vi "Default Settings.vi"(8 "error in (no error)":errorcluster, 11 "CAD Dispense in":refnum<class "CAD Dispense.lvclass">) -> (0 "error out":errorcluster, 3 "CAD Dispense out":refnum<class "CAD Dispense.lvclass">)   [LabVIEW 2020, in "CAD Dispense.lvclass"]
uses:
  CAD Dispense.lvclass
panel:
  # "This Routine does not Accept Settings"
  # "This Routine Does not Accept Settings"
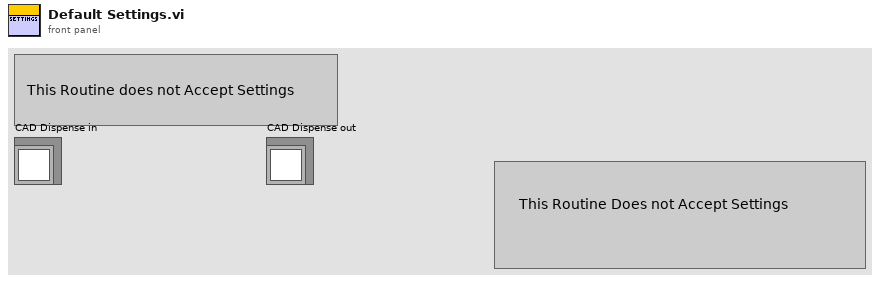
[diagram p1: front panel]
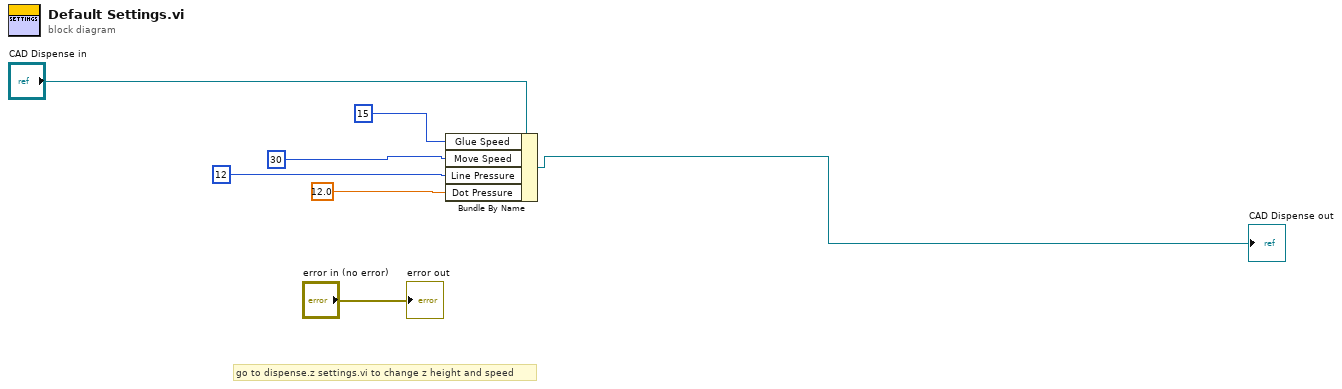
[diagram p0: block diagram]
diagram:
  # "go to dispense.z settings.vi to change z height and speed"
  n1 = Bundle By Name(cluster="CAD Dispense in", "Glue Speed"=15, "Move Speed"=30, "Line Pressure"=12, "Dot Pressure"=12.0) -> (→"CAD Dispense out":refnum<class "CAD Dispense.lvclass">)
  "error out" <- "error in (no error)"
